vi "Get_WavelengthPower.vi"(8 "error in (no error)":errorcluster, 10 "Index":u8, 11 "Abstract_Laser in":refnum<class "Abstract_Laser.lvclass">) -> (0 "error out":errorcluster, 1 "Power":dbl, 2 "Wavelength":dbl[unit], 3 "Abstract_Laser out":refnum<class "Abstract_Laser.lvclass">)   [LabVIEW 2020, in "Abstract_Laser.lvclass"]
uses:
  <instrlib>/Classes/Laser/Abstract_Laser/Abstract_Laser.lvclass
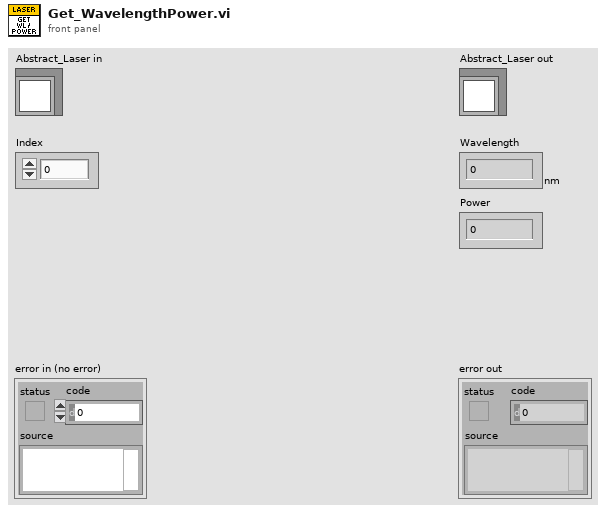
[diagram p1: front panel]
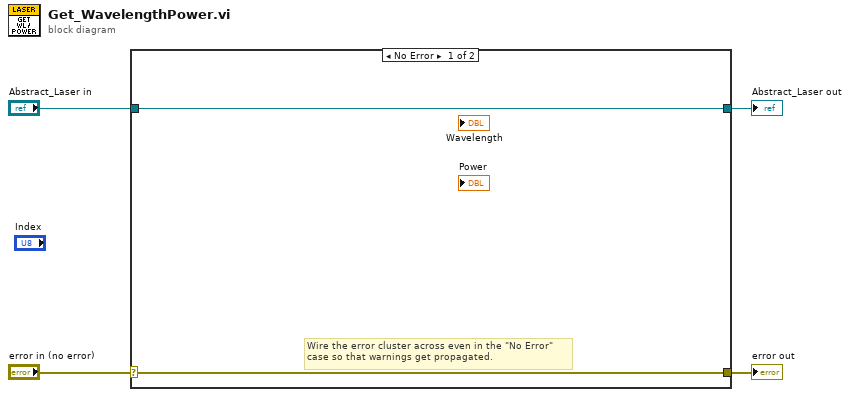
[diagram p0: block diagram]
diagram:
  n1 = case shown="No Error" "error in (no error)" {
    selector: "error in (no error)" -> [w5 w8]
    tunnel: [w5 w8] -> w3
    tunnel: [w6 w7] -> w1
    tunnel: "Abstract_Laser in" -> [w6 w7]
    frame No Error {
      # "Wire the error cluster across even in the \"No Error\"\ncase so that warnings get propagated."
    }
    frame Error {
    }
  }
  "error out" <- w3
  "Abstract_Laser out" <- w1
